vi "Initialize Connection with CD.vi"(8 "error in (no error)":errorcluster, 10 "Unit Computer Address":string, 11 "Custom Device Path":string) -> (0 "error out":errorcluster, 2 "Address Lookup Table":variant, 3 "connection info":T1)   [LabVIEW 2019, in "J1939 Host Automation API.lvlib"]
uses:
  J1939 Host Automation API.lvlib
  <vilib>/NI/STM/TCP/TCP Connection Info.ctl
  <vilib>/NI/STM/SubVIs/MetaDataElement.ctl
  Addon/Addon Shared/J1939 Addon Shared.lvlib
  <vilib>/NI/STM/NI STM.lvlib
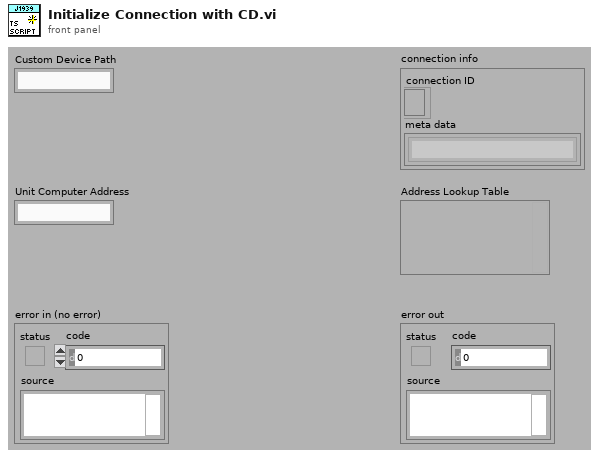
[diagram p1: front panel]
types:
  T1 = typedef "NI STM.lvlib/TCP Connection Info.ctl" = cluster{"connection ID":refnum<k5>, "meta data":T2[]}
  T2 = typedef "NI STM.lvlib/MetaDataElement.ctl" = string
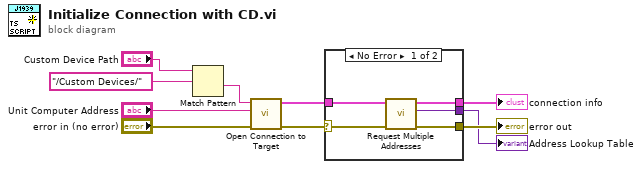
[diagram p0: block diagram]
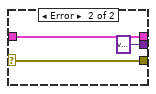
[diagram p2: hidden frame]
diagram:
  n1 = Match Pattern(string="Custom Device Path", regular expression="/Custom Devices/" ("Custom Device Path")) -> (after substring=w2:string)  [unwired: 1 in, 3 out]
  n2 = call "Open Connection to Target.vi"("error in (no error)"="error in (no error)", "IP Address"="Unit Computer Address", "TCP Service"=w2) -> ("error out"=w5:errorcluster, "connection info"=w7:T1)  [unwired: 7 in]
  n3 = case shown="No Error" w5 {
    selector: w5 -> [w14 w17]
    tunnel: w7 -> [w15 w18]
    tunnel: [w13 w17] -> w10
    tunnel: [w12 variant ("variant")] -> w8
    tunnel: [w11 w18] -> w9
    frame No Error {
      n4 = call "Request Multiple Addresses.vi"("error in (no error)"=w14, "connection info"=w15) -> ("error out"=w13:errorcluster, "variant"=w12:variant, "connection info"=w11:T1)  [unwired: 6 in, 1 out]
    }
    frame Error {
    }
  }
  "error out" <- w10
  "connection info" <- w9
  "Address Lookup Table" <- w8
